vi "solstis_initialize.vi"(10 "solstis port for remote interface":u16=39933, 11 "IP address of solstis(default 192.168.1.222)":string="192.168.1.222") -> (0 "error out":errorcluster, 3 "connection ID out":refnum<k5>)   [LabVIEW 2017]
panel:
  in  "Parameters":string[][](array[string])=[["\"ip_address\"", "\"192.168.1.110\""]]
  in  "Tx":i32=1
  in  "operation":string="\"start_link\""
  # "parameter values"
  # "to access solstis main console open web browser and type its IP address.\nusername: main  password: main\nnetwork settings under configure, make sure remote interface IP address matches\n lab PC IP address\n\nLab PC needs IPV4 static IP address 192.168.1.xxx, xxx is 3 numbers\nsubnet mask 255.255.255.0\ndefault gateway 192.168.1.1\nIn NI MAX set up a network device with the IP address of the Solstis and \nthe port listed in the solstis network settings for remote interface.\n\nIn solstis network settings give wavemeter same address as PC but a different port, \nmatching what is in the wavemeter server software."
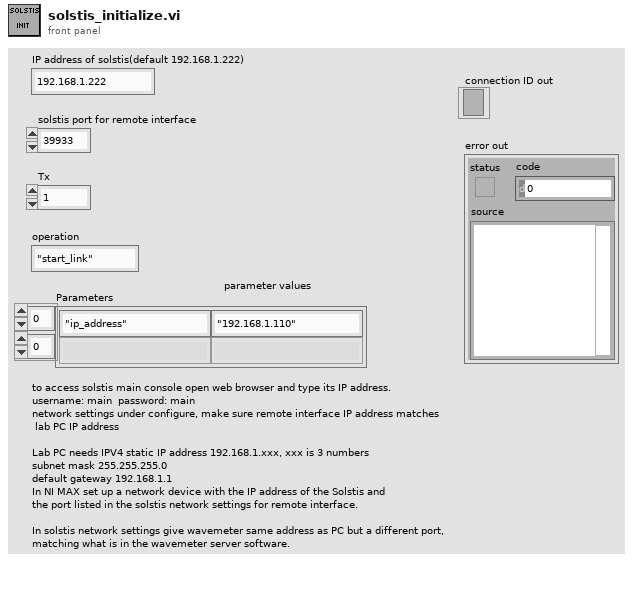
[diagram p1: front panel]
types:
  T1 = enum16{"Standard", "Buffered", "CRLF", "Immediate"}
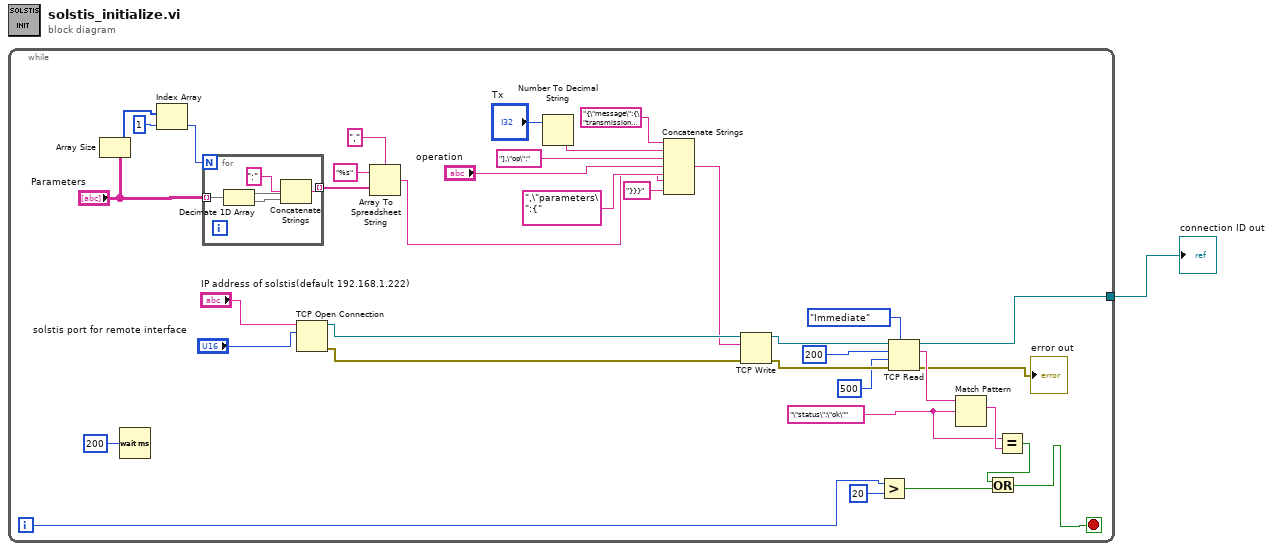
[diagram p0: block diagram]
diagram:
  n1 = while {
    tunnel: [w33] -> w1
    i -> [w6]
    stop <- w2 stop-if-true
    w8 = "\"status\":\"ok\"" ("regular expression")
    n2 = Array Size(array="Parameters") -> (size(s)=w17:i32[])
    n3 = Wait (ms)(milliseconds to wait=u32 200) -> ()  [unwired: 1 out]
    n4 = Index Array(array=w17, index=1) -> (element=w18:i32)
    n5 = for {
      N: w18 -> [_]
      tunnel: "Parameters" -> [w39] mode=indexing
      tunnel: [w38] -> w14 mode=indexing
      n6 = Decimate 1D Array(w39) -> (w41:string[], w40:string[])
      n7 = Concatenate Strings(w41, ":" ("string"), w40) -> (w38:string)
    }
    n8 = TCP Open Connection(address="IP address of solstis(default 192.168.1.222)", remote port or service name="solstis port for remote interface") -> (connection ID=w35:refnum<k5>, error out=w32:errorcluster)  [unwired: 1 in, 2 out]
    n9 = Array To Spreadsheet String(delimiter (Tab)=",", array=w14, 3:"%s" ("format string")) -> (spreadsheet string=w12:string)
    n10 = Number To Decimal String(number="Tx") -> (decimal integer string=w20:string)  [unwired: 1 out]
    n11 = Concatenate Strings("{\"message\":{\"transmission_id\":[" ("string"), w20, "],\"op\":" ("string"), "operation", ",\"parameters\":{" ("string"), w12, "}}}" ("string")) -> (w27:string)
    n12 = TCP Write(connection ID=w35, data in=w27, error in (no error)=w32) -> (connection ID out=w34:refnum<k5>, error out=w31:errorcluster)  [unwired: 2 out]
    n13 = Greater?(x=w6, y=20) -> (0:w4:bool)
    n14 = TCP Read(connection ID=w34, bytes to read=200, error in (no error)=w31, 7:T1."Immediate" ("mode (standard)"), 9:500 ("timeout ms (25000)")) -> (connection ID out=w33:refnum<k5>, data out=w10:string, error out=→"error out":errorcluster)
    n15 = Match Pattern(string=w10, regular expression=w8) -> (match substring=w9:string)  [unwired: 4 out]
    n16 = Equal?(x=w8, y=w9) -> (x = y?=w3:bool)
    n17 = Or(x=w3, y=w4) -> (x .or. y?=w2:bool)
  }
  "connection ID out" <- w1
